vi "Configure TS DACs.vi"(8 "error in":errorcluster, 11 "DeepU Test Stand in":refnum<class "DeepU Test Stand.lvclass">) -> (0 "error out":errorcluster, 3 "DeepU Test Stand out":refnum<class "DeepU Test Stand.lvclass">)   [LabVIEW 2019, in "Test Stands.lvlib" / "DeepU Test Stand.lvclass"]
uses:
  DeepU Test Stand.lvclass
  DeepU Test Stand.lvclass/DeepU Test Stand.ctl
  <vilib>/DAQmx/create/scale.llb/DAQmx Create Scale (Map Ranges).vi
  <vilib>/DAQmx/create/channels.llb/DAQmx Create Channel (AI-Current-Basic).vi
  <vilib>/DAQmx/create/channels.llb/DAQmx Create Channel (DO-Digital Output).vi
  <resource>/objmgr/daqmx.rc
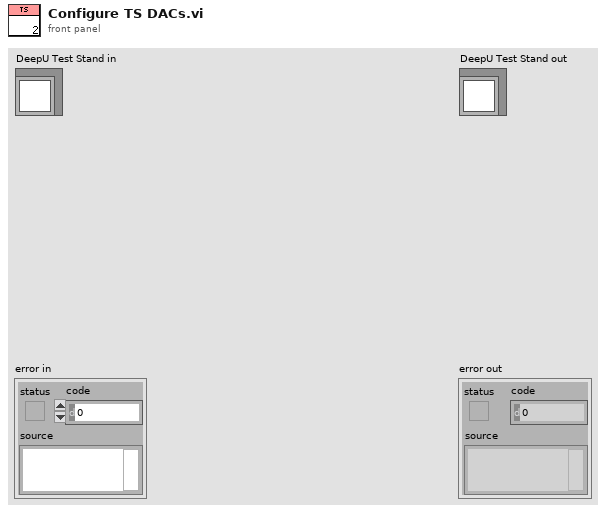
[diagram p1: front panel]
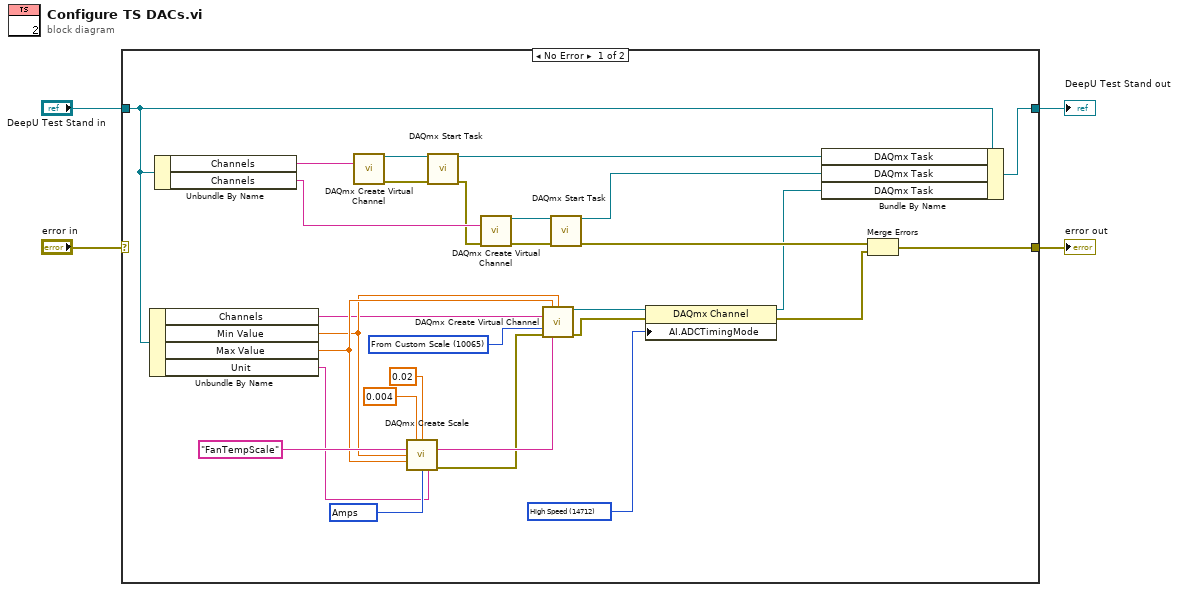
[diagram p0: block diagram]
diagram:
  n1 = case shown="No Error" "error in" {
    selector: "error in" -> [_ w35]
    tunnel: [w21 w35] -> w3
    tunnel: [w33 w34] -> w1
    tunnel: "DeepU Test Stand in" -> [w31 w34]
    frame No Error {
      w8 = 14712 items=["Automatic"=16097, "High Resolution"=10195, "High Speed"=14712, "Best 50 Hz Rejection"=14713, "Best 60 Hz Rejection"=14714, "Custom"=10137] ("AI.ADCTimingMode")
      w25 = 10342 items=["Volts"=10348, "Amps"=10342, "Deg F"=10144, "Deg C"=10143, "Deg R"=10145, "Kelvins"=10325, "Strain"=10299, "Ohms"=10384, "Hz"=10373, "Seconds"=10364, "Meters"=10219, "Inches"=10379, "Degrees"=10146, "Radians"=10273, "Ticks"=10304, "g"=10186, "m/s^2"=12470, "m/s"=15959, "in/s"=15960, "Pascals"=10081, "Newtons"=15875, "Pounds"=15876, "kgf"=15877, "psi"=15879, "bar"=15880, "Nm"=15881, "oz-in"=15882, "lb-in"=15883, "lb-ft"=15884, "Volts/Volt"=15896, "mVolts/Volt"=15897, "pCoulombs"=16103, "Coulombs"=16102, "From TEDS"=12516] ("pre-scaled units")
      w26 = 10065 items=["Amps"=10342, "From Custom Scale"=10065] ("units")
      n2 = Unbundle By Name(w31) -> ("Channels"=w18:string, "Min Value"=w23:dbl, "Max Value"=w24:dbl, "Unit"=w20:string)
      n3 = Unbundle By Name(w31) -> ("Channels"=w19:string, "Channels"=w32:string)
      n4 = call-poly <vilib>:"DAQmx Create Virtual Channel.vi"("lines"=w19) -> ("task out"=w17:refnum<k21>, "error out"=w16:errorcluster)  [unwired: 13 in]
      n5 = call-poly <vilib>:"DAQmx Create Scale.vi"("pre-scaled minimum"=0.004, "pre-scaled maximum"=0.02, "name"="FanTempScale", "scaled minimum"=w23, "scaled maximum"=w24, "pre-scaled units"=w25, "scaled units"=w20) -> ("scale out"=w27:tag, "error out"=w22:errorcluster)  [unwired: 7 in]
      n6 = call <vilib>:"DAQmx Start Task.vi"("task/channels in"=w17, "error in"=w16) -> ("task out"=w15:refnum<k21>, "error out"=w14:errorcluster)  [unwired: 12 in]
      n7 = call-poly <vilib>:"DAQmx Create Virtual Channel.vi"("lines"=w32, "error in"=w14) -> ("task out"=w12:refnum<k21>, "error out"=w13:errorcluster)  [unwired: 12 in]
      n8 = call-poly <vilib>:"DAQmx Create Virtual Channel.vi"("maximum value"=w24, "minimum value"=w23, "physical channels"=w18, "units"=w26, "error in"=w22, "custom scale name"=w27) -> ("task out"=w9:refnum<k21>, "error out"=w6:errorcluster)  [unwired: 8 in]
      n9 = call <vilib>:"DAQmx Start Task.vi"("task/channels in"=w12, "error in"=w13) -> ("task out"=w11:refnum<k21>, "error out"=w10:errorcluster)  [unwired: 12 in]
      n10 = property class="DAQmx Channel"(reference=w9, error in=w6, "AI.ADCTimingMode"=w8) -> (reference out=w7:refnum<k21>, error out=w5:errorcluster)
      n11 = Bundle By Name(cluster=w31, "DAQmx Task"=w15, "DAQmx Task"=w11, "DAQmx Task"=w7) -> (w33:refnum<class "DeepU Test Stand.lvclass">)
      n12 = Merge Errors(w10, w5) -> (w21:errorcluster)
    }
    frame Error {
    }
  }
  "error out" <- w3
  "DeepU Test Stand out" <- w1
